vi "Get Node Data (String).vi"(3 "element id":i32, 5 "level":i32, 6 "Attribute? (F=Entity)":bool, 7 "contains raw xml":bool, 8 "error in (no error)":errorcluster, 9 "Default Value (\"\")":string, 10 "Attribute Name":string, 11 "xml":T1) -> (0 "error out":errorcluster, 1 "Data Value":string, 2 "found?":bool)   [LabVIEW 2013]
doc: "Returns the <B>Data Value</B> (text or cdata-section) of <B>Node</B>. If none is found, <B>Default Value</B> will be used."
uses:
  Fast Parser/XML Structure - Cluster.ctl
  Fast Parser/XML Tag Type - Enum.ctl
panel:
  # "Copyright © 2006 James Kring, Inc. All rights reserved.\n\nAuthor: Jim Kring <jim.kring@jameskring.com>\n\nThis library is provided \"AS IS\" , WITHOUT WARRANTIES OR \nCONDITIONS OF ANY KIND, either express or implied.\n\nJames Kring, Inc. -- http://www.jameskring.com"
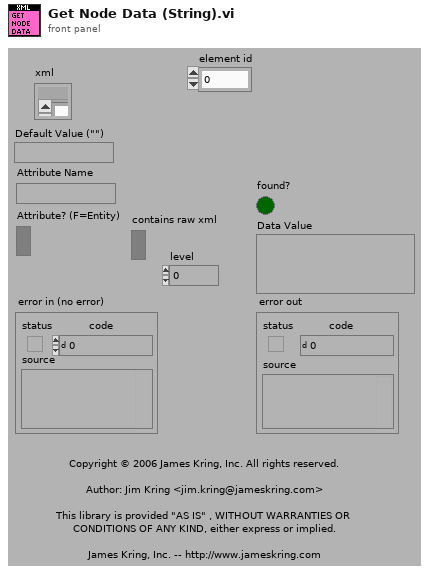
[diagram p1: front panel]
types:
  T1 = typedef "XML Structure - Cluster.ctl" = cluster{"tags":string[], "tag names":string[], "tag type":T2[], "offset":i32[], "close tag index":i32[], "xml":string, "Children":cluster{"children":i32[]}[], "parent index":i32[]}
  T2 = typedef "XML Tag Type - Enum.ctl" = enum16{"start tag", "empty tag", "end tag"}
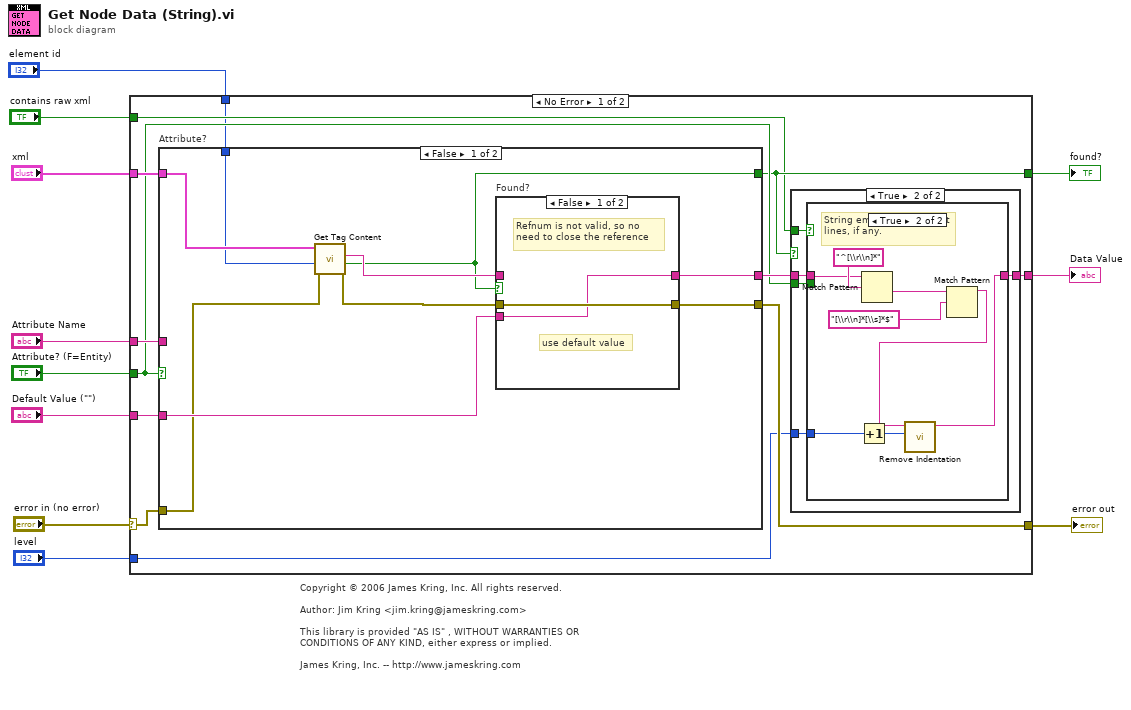
[diagram p0: block diagram]
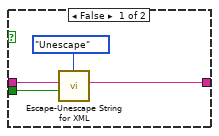
[diagram p3: hidden frame]
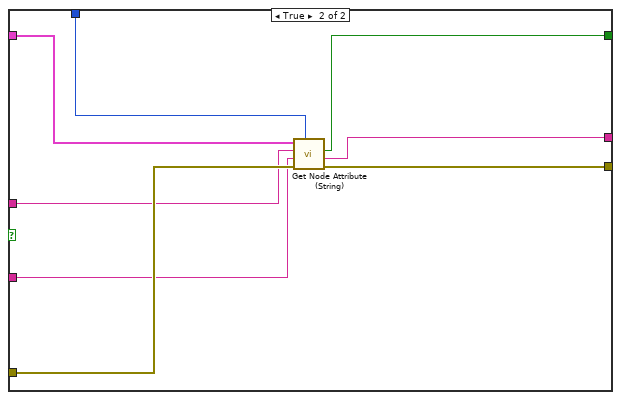
[diagram p5: hidden frame]
diagram:
  # "Copyright © 2006 James Kring, Inc. All rights reserved.\n\nAuthor: Jim Kring <jim.kring@jameskring.com>\n\nThis library is provided \"AS IS\" , WITHOUT WARRANTIES OR \nCONDITIONS OF ANY KIND, either express or implied.\n\nJames Kring, Inc. -- http://www.jameskring.com"
  n1 = case shown="No Error" "error in (no error)" {
    selector: "error in (no error)" -> [w23 w63]
    tunnel: "xml" -> [w20 _]
    tunnel: [w17 _] -> w10
    tunnel: [w21 w63] -> w11
    tunnel: [w15 _] -> w7
    tunnel: "Default Value (\"\")" -> [w22 _]
    tunnel: "Attribute? (F=Entity)" -> [w16 _]
    tunnel: "Attribute Name" -> [w19 _]
    tunnel: "contains raw xml" -> [w14 _]
    tunnel: "level" -> [w13 _]
    tunnel: "element id" -> [w12 _]
    frame No Error {
      n2 = case "Attribute?" shown="False" w16 {
        tunnel: w23 -> [w44 w62]
        tunnel: w22 -> [w50 w58]
        tunnel: [w49 w61] -> w21
        tunnel: [w48 w57] -> w18
        tunnel: [w42 w56] -> w15
        tunnel: w20 -> [w47 w60]
        tunnel: w19 -> [_ w59]
        tunnel: w12 -> [w46 w55]
        frame False {
          n3 = call "Get Tag Content.vi"("error in (no error)"=w44, "tag index"=w46, "xml in"=w47) -> ("error out"=w43:errorcluster, "found?"=w42:bool, "element content"=w45:string)  [unwired: 5 in, 1 out]
          n4 = case "Found?" shown="False" w42 {
            tunnel: [w51 w53] -> w48
            tunnel: w43 -> [w52 w54]
            tunnel: [w52 w54] -> w49
            tunnel: w45 -> [_ w53]
            tunnel: w50 -> [w51 _]
            frame False {
              # "use default value"
              # "Refnum is not valid, so no need to close the reference"
            }
            frame True {
            }
          }
        }
        frame True {
          n5 = call "Get Node Attribute (String).vi"("element id"=w55, "error in (no error)"=w62, "Default Value (\"\")"=w58, "Attribute Name"=w59, "xml"=w60) -> ("error out"=w61:errorcluster, "Attribute Value"=w57:string, "found?"=w56:bool)  [unwired: 4 in]
        }
      }
      n6 = case shown="True" w15 {
        tunnel: w18 -> [w24 w29]
        tunnel: [w24 w28] -> w17
        tunnel: w16 -> [_ w27]
        tunnel: w14 -> [_ w26]
        tunnel: w13 -> [_ w25]
        frame False {
        }
        frame True {
          n7 = case shown="True" w26 {
            tunnel: w29 -> [w32 w39]
            tunnel: [w31 w41] -> w28
            tunnel: w27 -> [w30 _]
            tunnel: w25 -> [_ w35]
            frame False {
              n8 = call "Escape-Unescape String for XML.vi"("attribute? (F: entity)"=w30, "String"=w32, "Action (Escape)"=enum16{"Escape", "Unescape"}."Unescape") -> ("String out"=w31:string)  [unwired: 8 in]
            }
            frame True {
              # "String empty first and last lines, if any."
              n9 = Increment(x=w35) -> (x+1=w34:i32)
              n10 = Match Pattern(string=w39, regular expression="^[\\r\\n]*" ("string")) -> (after substring=w38:string)  [unwired: 1 in, 3 out]
              n11 = Match Pattern(string=w38, regular expression="[\\r\\n]*[\\s]*$" ("string")) -> (before substring=w37:string)  [unwired: 1 in, 3 out]
              n12 = call "Remove Indentation.vi"("levels to remove"=w34, "String in"=w37) -> ("String"=w41:string)  [unwired: 9 in]
            }
          }
        }
      }
    }
    frame Error {
    }
  }
  "error out" <- w11
  "Data Value" <- w10
  "found?" <- w7
